vi "Constants.vi"() -> ()   [LabVIEW 2021, in "G5 Regatron Custom Device Shared.lvlib"]
doc: "Use this Global VI to access the GUIDs assigned to the page resources of the Custom Device."
uses:
  G5 Regatron Custom Device Shared.lvlib
panel:
  in  "Tab Control":enum32{"GUIDs", "Constants", "Properties"}(tab)
  in  "G5 Regatron Custom Device":string="6c2b54bf-7fd6-4da4-9695-684477d5d7ed"
  in  "IP Address":string
  in  "Compiled.Settings":string="Compiled.Settings"
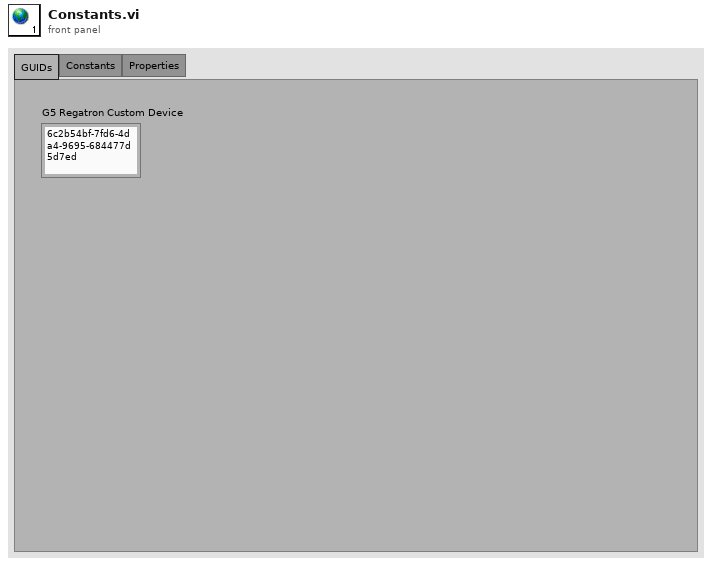
[diagram p1: front panel]
diagram:
